vi "Sort Keys.vi"(8 "error in":errorcluster, 11 "Refnum in":T2) -> (0 "error out":errorcluster, 2 "Sorted Data":T1, 3 "Refnum out":T2)   [LabVIEW 2012]
uses:
  <vilib>/Utility/config.llb/Config Data RefNum.ctl
  <userlib>/_OpenG.lib/array/array.llb/Sort 1D Array (DBL)__ogtk.vi
  <vilib>/Utility/config.llb/Read Key (Double).vi
  <vilib>/Utility/config.llb/Read Key (String).vi
  <vilib>/Utility/config.llb/NI_LVConfig.lvlib
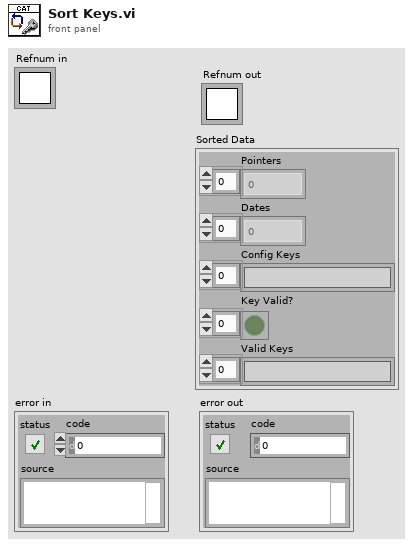
[diagram p1: front panel]
types:
  T1 = cluster{"Pointers":i32[], "Dates":dbl[], "Config Keys":string[], "Key Valid?":bool[], "Valid Keys":string[]}
  T2 = typedef "NI_LVConfig.lvlib/Config Data RefNum.ctl" = refnum<k1>
  T3 = cluster{"Pointers":i32[], "Dates":dbl[], "Keys":string[], "Key Valid?":bool[], string[]}
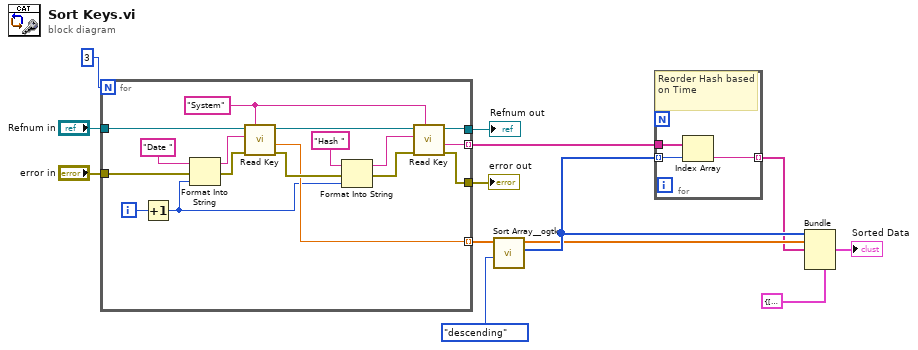
[diagram p0: block diagram]
diagram:
  n1 = for {
    N: 3 -> [_]
    tunnel: "Refnum in" -> [w22]
    tunnel: [w21] -> w11 mode=indexing
    tunnel: [w20] -> w12 mode=indexing
    tunnel: [w19] -> w9
    tunnel: [w18] -> w8
    tunnel: "error in" -> [w17]
    i -> [w16]
    w14 = "System" ("section")
    n2 = Increment(x=w16) -> (x+1=w15:i32)
    n3 = Format Into String(initial string="Date " ("key"), error in=w17, w15) -> (resulting string=w28:string, error out=w27:errorcluster)  [unwired: 1 in]
    n4 = call-poly <vilib>:"Read Key.vi"("section"=w14, "error in (no error)"=w27, "key"=w28, "refnum"=w22) -> ("error out"=w26:errorcluster, "value"=w20:dbl, "refnum out"=w30:T2)  [unwired: 4 in, 1 out]
    n5 = Format Into String(initial string="Hash " ("key"), error in=w26, w15) -> (resulting string=w29:string, error out=w25:errorcluster)  [unwired: 1 in]
    n6 = call-poly <vilib>:"Read Key.vi"("section"=w14, "error in (no error)"=w25, "key"=w29, "refnum"=w30) -> ("error out"=w18:errorcluster, "value"=w21:string, "refnum out"=w19:T2)  [unwired: 4 in, 1 out]
  }
  "Refnum out" <- w9
  "error out" <- w8
  n7 = call-poly <userlib>:"Sort Array__ogtk.vi"("Order"=enum16{"ascending", "descending"}."descending", "Array in"=w12) -> ("Sorted Pointers"=w5:i32[], "Sorted Array out"=w4:dbl[])  [unwired: 8 in]
  n8 = for {
    tunnel: w5 -> [w32] mode=indexing
    tunnel: w11 -> [w33]
    tunnel: [w31] -> w3 mode=indexing
    # "Reorder Hash based on Time"
    n9 = Index Array(array=w33, index=w32) -> (element=w31:string)
  }
  n10 = Bundle(cluster=T3 {"Pointers"=[], "Dates"=[], "Keys"=[], "Key Valid?"=[], []} ("Sorted Data"), "Pointers"=w5, "Dates"=w4, "Keys"=w3) -> (→"Sorted Data":T3)  [unwired: 2 in]
